vi "get_image_imaq.vi"(8 "error in":errorcluster, 9 "Image Resource In":T2, 10 "fmt":T1(ring), 11 "index":i32) -> (0 "error out":errorcluster, 1 "Image Resource Out":T2)   [LabVIEW 2017, in "libfreenect.lvlib"]
uses:
  libfreenect.lvlib
  <vilib>/vision/Image Controls.llb/IMAQ Image.ctl
  <vilib>/vision/NI_Vision_Development_Module.lvlib
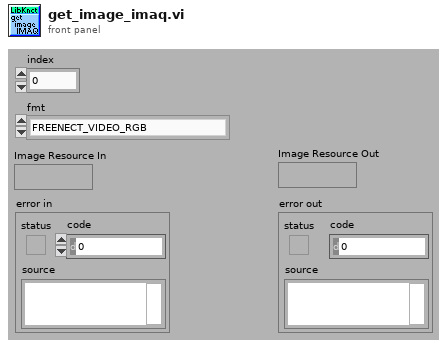
[diagram p1: front panel]
types:
  T1 = enum16{"FREENECT_VIDEO_RGB", "FREENECT_VIDEO_BAYER", "FREENECT_VIDEO_IR_8BIT", "FREENECT_VIDEO_IR_10BIT", "FREENECT_VIDEO_IR_10BIT_PACKED", "FREENECT_VIDEO_YUB_RGB", "FREENECT_VIDEO_YUB_RAW"}
  T2 = typedef "IMAQ Image.ctl" = refnum<image>
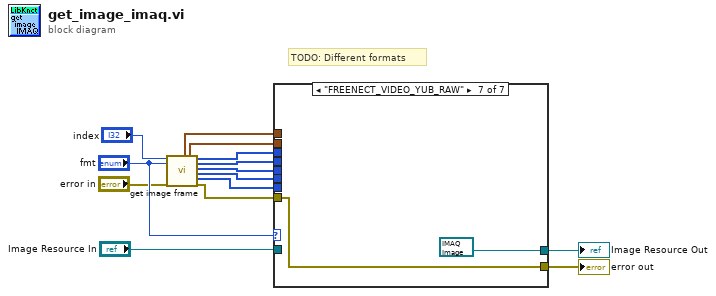
[diagram p0: block diagram]
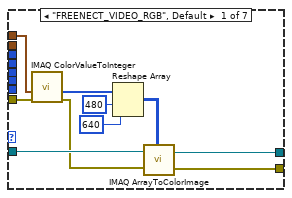
[diagram p2: hidden frame]
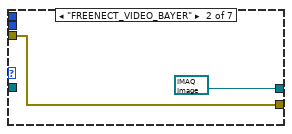
[diagram p3: hidden frame]
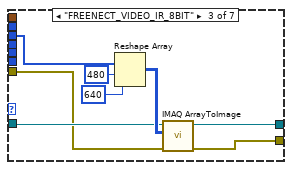
[diagram p4: hidden frame]
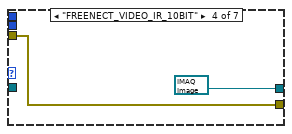
[diagram p5: hidden frame]
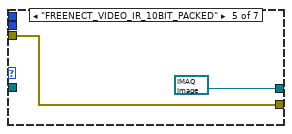
[diagram p6: hidden frame]
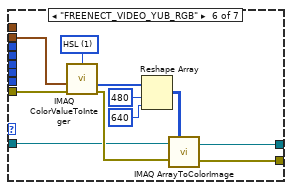
[diagram p7: hidden frame]
diagram:
  # "TODO: Different formats"
  n1 = call "get image frame.vi"("index"="index", "fmt"="fmt", "error in (no error)"="error in") -> ("RGB Array"=w8:cluster{"R":u8, "G":u8, "B":u8}[], "YUB RGB Array"=w7:cluster{"R":u8, "G":u8, "B":u8}[], "Bayer Array"=w6:u8[], "IR 8Bit Array"=w5:u8[], "IR 10Bit Array"=w4:u16[], "YUB RAW Array"=w3:u16[], "IR 10Bit Packed Array"=w2:u8[], "error out"=w1:errorcluster)  [unwired: 9 out]
  n2 = case shown="\"FREENECT_VIDEO_YUB_RAW\"" "fmt" {
    tunnel: [w21 T2 refnum ("Image Out") w32 T2 refnum ("Image Out") T2 refnum ("Image Out") w40 T2 refnum ("Image Out")] -> w13
    tunnel: w8 -> [w18 _ _ _ _ _ _]
    tunnel: "Image Resource In" -> [w20 _ w29 _ _ w42 _]
    tunnel: [w19 w25 w30 w35 w37 w39 w50] -> w12
    tunnel: w1 -> [w16 w25 w28 w35 w37 w41 w50]
    tunnel: w7 -> [_ _ _ _ _ w43 _]
    tunnel: w6 -> [_ _ _ _ _ _ _]
    tunnel: w5 -> [_ _ w27 _ _ _ _]
    tunnel: w4 -> [_ _ _ _ _ _ _]
    tunnel: w3 -> [_ _ _ _ _ _ _]
    tunnel: w2 -> [_ _ _ _ _ _ _]
    frame "FREENECT_VIDEO_RGB", Default {
      n3 = call "IMAQ ColorValueToInteger"("error in (no error)"=w16, "1D Color value array"=w18) -> ("1D U32 array"=w17:u32[], "error out"=w15:errorcluster)  [unwired: 3 in, 2 out]
      n4 = Reshape Array(w17, 480 ("dimension size"), 640 ("dimension size")) -> (w22:u32[][])
      n5 = call "IMAQ ArrayToColorImage"("Image Pixels (U32)"=w22, "Image"=w20, "error in (no error)"=w15) -> ("Image Out"=w21:T2, "error out"=w19:errorcluster)  [unwired: 1 in, 1 out]
    }
    frame "FREENECT_VIDEO_BAYER" {
    }
    frame "FREENECT_VIDEO_IR_8BIT" {
      n6 = Reshape Array(w27, 480 ("dimension size"), 640 ("dimension size")) -> (w31:u8[][])
      n7 = call "IMAQ ArrayToImage"("error in (no error)"=w28, "Image Pixels (U8)"=w31, "Image"=w29) -> ("error out"=w30:errorcluster, "Image Out"=w32:T2)  [unwired: 3 in, 4 out]
    }
    frame "FREENECT_VIDEO_IR_10BIT" {
    }
    frame "FREENECT_VIDEO_IR_10BIT_PACKED" {
    }
    frame "FREENECT_VIDEO_YUB_RGB" {
      w44 = u16 1 items=["RGB", "HSL", "HSV", "HSI"] ("Color Mode")
      n8 = call "IMAQ ColorValueToInteger"("error in (no error)"=w41, "1D Color value array"=w43, "Color Mode"=w44) -> ("1D U32 array"=w48:u32[], "error out"=w49:errorcluster)  [unwired: 2 in, 2 out]
      n9 = Reshape Array(w48, 480 ("dimension size"), 640 ("dimension size")) -> (w47:u32[][])
      n10 = call "IMAQ ArrayToColorImage"("Image Pixels (U32)"=w47, "Image"=w42, "error in (no error)"=w49) -> ("Image Out"=w40:T2, "error out"=w39:errorcluster)  [unwired: 1 in, 1 out]
    }
    frame "FREENECT_VIDEO_YUB_RAW" {
    }
  }
  "Image Resource Out" <- w13
  "error out" <- w12
